vi "code.vi"() -> ()   [LabVIEW 2022 SP3]
uses:
  <vilib>/Instr/_visa.llb/VISA Configure Serial Port (Instr).vi
panel:
  out "Gauge 2":cluster{dbl, dbl}(knob)={1.5203080545981167, 1.5203080545981167} caption="Gauge" scale=0.0..8.0 scale format="%01d"
  in  "stop":bool
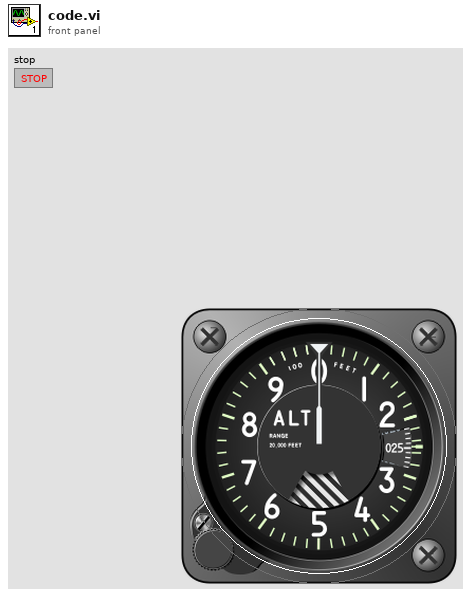
[diagram p1: front panel]
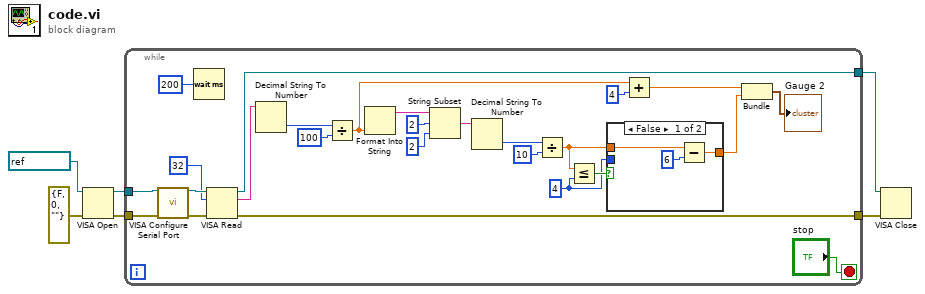
[diagram p0: block diagram]
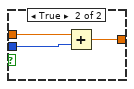
[diagram p2: hidden frame]
diagram:
  n1 = VISA Open(error in (no error)=errorcluster {"status"=FALSE, "code"=0, "source"=""}, VISA resource name=refnum<visa-resource-name> "COM8") -> (VISA resource name=w2:refnum<visa-resource-name>, error out=w3:errorcluster)  [unwired: 3 in]
  n2 = while {
    tunnel: [w30] -> w6
    tunnel: [w29] -> w5
    tunnel: w3 -> [w25]
    tunnel: w2 -> [w24]
    stop <- "stop" stop-if-true
    w10 = 4
    n3 = call-poly "VISA Configure Serial Port"("VISA resource name"=w24, "error in (no error)"=w25) -> ("VISA resource name out"=w31:refnum<visa-resource-name>, "error out"=w32:errorcluster)  [unwired: 12 in]
    n4 = Wait (ms)(milliseconds to wait=u32 200) -> ()  [unwired: 1 out]
    n5 = VISA Read(VISA resource name=w31, byte count=u32 32, error in (no error)=w32) -> (VISA resource name out=w30:refnum<visa-resource-name>, read buffer=w23:string, error out=w29:errorcluster)  [unwired: 1 out]
    n6 = Decimal String To Number(string=w23) -> (number=w20:i32)  [unwired: 2 in, 1 out]
    n7 = Divide(x=w20, y=100) -> (x/y=w19:dbl)
    n8 = Format Into String(w19) -> (resulting string=w18:string)  [unwired: 3 in, 1 out]
    n9 = String Subset(string=w18, offset (0)=2, length (rest)=2 ("length (rest)")) -> (substring=w15:string)
    n10 = Decimal String To Number(string=w15) -> (number=w14:i32)  [unwired: 2 in, 1 out]
    n11 = Divide(x=w14, y=10) -> (x/y=w11:dbl)
    n12 = Less Or Equal?(x=w11, y=w10) -> (x <= y?=w12:bool)
    n13 = case shown="False" w12 {
      tunnel: w11 -> [w35 w38]
      tunnel: w10 -> [_ w37]
      tunnel: [w34 w36] -> w8
      frame False {
        n14 = Subtract(x=w35, y=6) -> (x-y=w34:dbl)
      }
      frame True {
        n15 = Add(x=w38, y=w37) -> (x+y=w36:dbl)
      }
    }
    n16 = Add(x=w19, y=4) -> (x+y=w9:dbl)
    n17 = Bundle(w9, w8) -> (→"Gauge 2":cluster{dbl, dbl})  [unwired: 1 in]
  }
  n18 = VISA Close(VISA resource name=w6, error in (no error)=w5) -> ()  [unwired: 1 out]
